vi "Update Message.vi"(4 "Pop Receipt":string, 6 "Message ID":string, 7 "Visibility Timeout (0 seconds)":i32, 8 "error in (no error)":errorcluster, 9 "Message":string, 10 "Queue":string, 11 "Azure Session in":refnum<class "Session.lvclass">) -> (0 "error out":errorcluster, 3 "Azure Session out":refnum<class "Session.lvclass">)   [LabVIEW 2015, in "NI_Azure_Queue.lvlib"]
doc: "Updates the visibility timeout of a message and/or the message contents."
uses:
  NI_Azure_Queue.lvlib
  Core/Session/Session.lvclass
  Core/Name Value Pair.ctl
  Core/Session/Session.lvclass/Session.ctl
  Core/Session/Write HTTP Verb.vi
  Core/Session/Write URL Suffix.vi
  Core/Session/Write Request body.vi
  Core/Session/Write Request Parameters.vi
  Core/NI_Azure_Core.lvlib
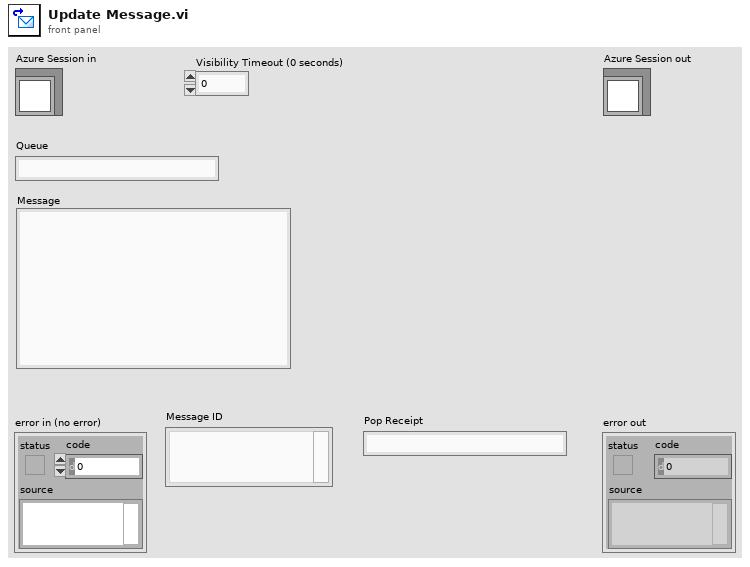
[diagram p1: front panel]
types:
  T1 = typedef "NI_Azure_Core.lvlib/Name Value Pair.ctl" = cluster{"name":string, "value":string}
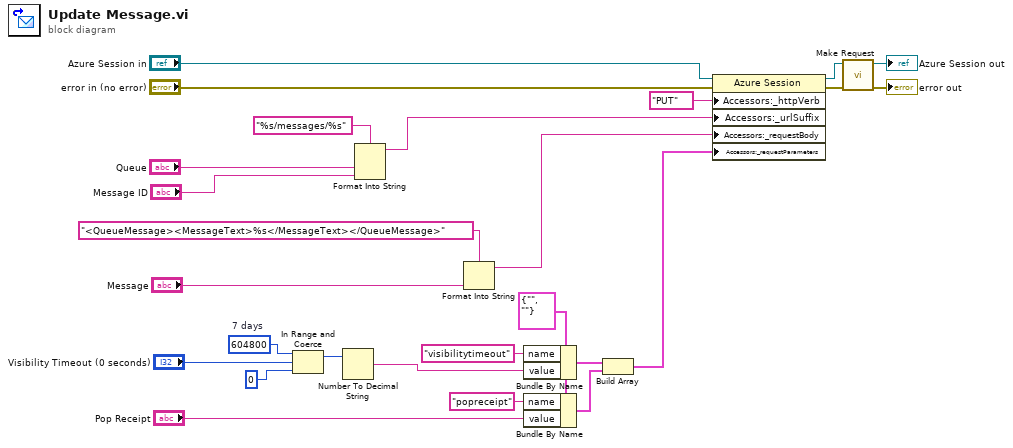
[diagram p0: block diagram]
diagram:
  w4 = u32 604800  # 7 days
  w12 = T1 {"name"="", "value"=""} ("Name Value Pair")
  n1 = In Range and Coerce(upper limit=w4, x="Visibility Timeout (0 seconds)", lower limit=u32 0) -> (coerced(x)=w3:u32)  [unwired: 1 out]
  n2 = Number To Decimal String(number=w3) -> (decimal integer string=w1:string)  [unwired: 1 in]
  n3 = Format Into String(format string="%s/messages/%s", "Queue", "Message ID") -> (resulting string=w17:string)  [unwired: 2 in, 1 out]
  n4 = Format Into String(format string="<QueueMessage><MessageText>%s</MessageText></QueueMessage>", "Message") -> (resulting string=w15:string)  [unwired: 2 in, 1 out]
  n5 = Bundle By Name(cluster=w12, "name"="visibilitytimeout", "value"=w1) -> (w13:T1)
  n6 = Bundle By Name(cluster=w12, "name"="popreceipt", "value"="Pop Receipt") -> (w11:T1)
  n7 = Build Array(w13, w11) -> (w8:T1[])
  n8 = property class="Azure Session"(reference="Azure Session in", error in="error in (no error)", "Accessors:_httpVerb"="PUT" ("HTTP-Verb"), "Accessors:_urlSuffix"=w17, "Accessors:_requestBody"=w15, "Accessors:_requestParameters"=w8) -> (reference out=w21:refnum<class "Session.lvclass">, error out=w19:errorcluster)
  n9 = call "Make Request.vi"("error in (no error)"=w19, "Session in"=w21) -> ("error out"=→"error out":errorcluster, "Session out"=→"Azure Session out":refnum<class "Session.lvclass">)  [unwired: 7 in, 1 out]
